vi "Tosca-Init Histogram.vi"(0 "Histogram":refnum<vi>, 7 "Results":T1[](array[typedef]), 11 "error in (no error)":errorcluster) -> (15 "error out":errorcluster)   [LabVIEW 2020]
uses:
  Classes/Parameters/Histogram Data.ctl
  <vilib>/Analysis/baseanly.llb/Mean (DBL).vi
  <vilib>/Analysis/NI_AALBase.lvlib
  Classes/Parameters/Parameters.lvclass
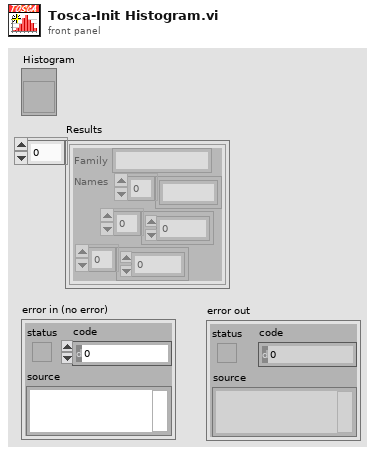
[diagram p1: front panel]
types:
  T1 = typedef "Parameters.lvclass/Histogram Data.ctl" = cluster{"Family":string, "Names":string[], "Colors":u32[], "N":i32[]}
  T2 = cluster{"Name":string, "Color":u32, "Style":u8, "Point Style":u8, "Name Visible":bool, "Allow Drag":bool, "Annotation Mode":u32, "Plot":i32, "Index":i32, "Position":cluster{"X":dbl, "Y":dbl}, "X Scale":u32, "Y Scale":u32, "Show Arrow":bool, "Lock Name":bool, "Plot Area":i32, "Label Offset":cluster{"X":dbl, "Y":dbl}}
  T3 = cluster{"Name":string, "Color":u32, "Style":u8, "Point Style":u8, "Name Visible":bool, "Allow Drag":bool, "Annotation Mode":u32, "Plot":i32, "Index":i32, "Position":cluster{"X":dbl, "Y":dbl}, "X Scale":u32, "Y Scale":u32, "Show Arrow":bool, "Lock Name":bool, "Plot Area":i32, "Label Offset":cluster{"X":dbl, "Y":dbl}}[]
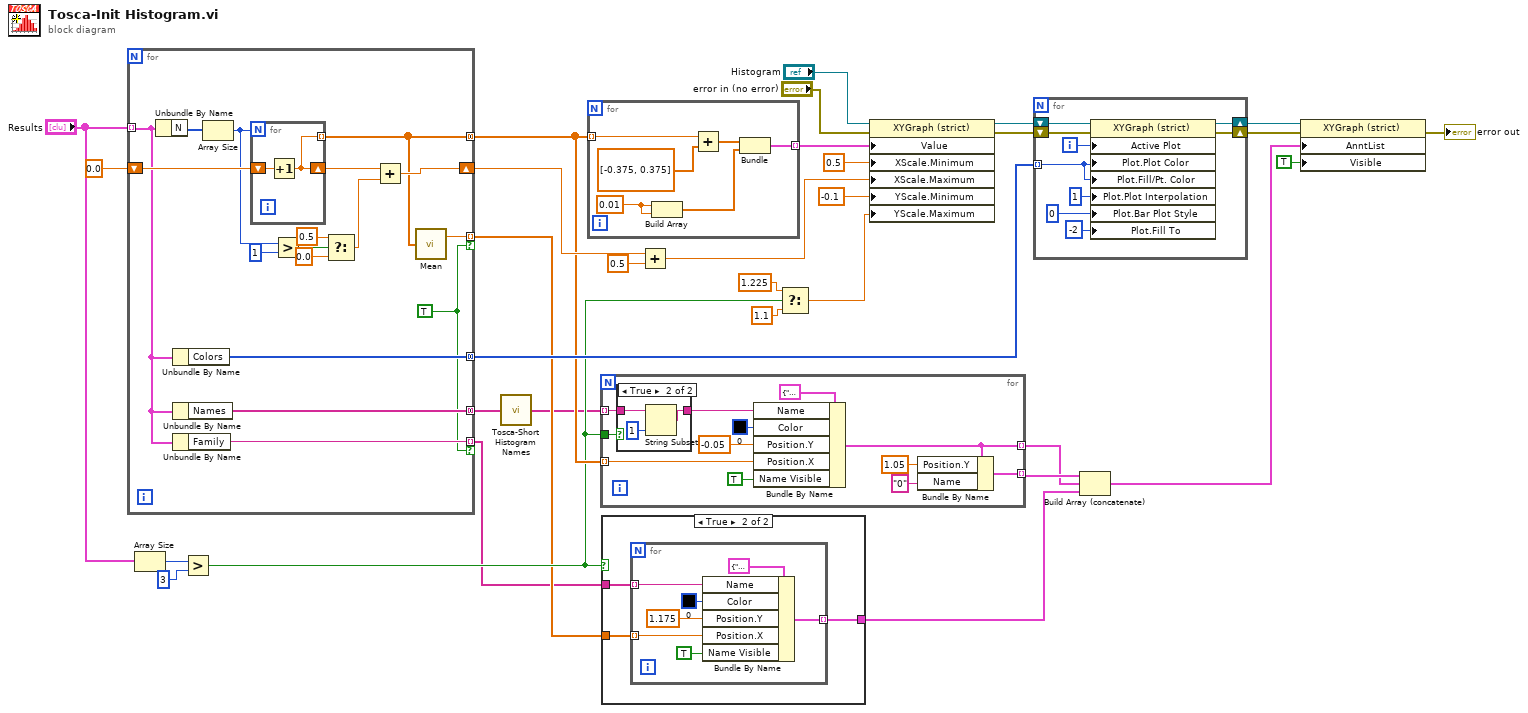
[diagram p0: block diagram]
diagram:
  n1 = for {
    tunnel: "Results" -> [w35] mode=indexing
    shift-right: [w47] -> w26
    shift-left: 0.0 -> [w49]
    tunnel: [w39] -> w15 mode=concatenating
    tunnel: [w36] -> w27 mode=concatenating
    tunnel: [w34] -> w2 mode=concatenating
    tunnel: [w37] -> w5 mode=indexing if=w33
    tunnel: [w38] -> w6 mode=indexing if=w33
    w33 = TRUE
    n2 = Unbundle By Name(w35) -> ("N"=w41:i32[])
    n3 = Unbundle By Name(w35) -> ("Colors"=w36:u32[])
    n4 = Unbundle By Name(w35) -> ("Names"=w34:string[])
    n5 = Unbundle By Name(w35) -> ("Family"=w37:string)
    n6 = Array Size(array=w41) -> (size(s)=w40:i32)
    n7 = for {
      N: w40 -> [_]
      tunnel: [w50] -> w39 mode=indexing
      shift-right: [w50] -> w48
      shift-left: w49 -> [w51]
      n8 = Increment(x=w51) -> (x+1=w50:dbl)
    }
    n9 = Greater?(x=w40, y=1) -> (0:w45:bool)
    n10 = Select(t=0.5, s=w45, f=0.0) -> (s? t:f=w43:dbl)
    n11 = Add(x=w48, y=w43) -> (x+y=w47:dbl)
    n12 = call-poly <vilib>:"Mean.vi"("X"=w39) -> ("mean"=w38:dbl)  [unwired: 1 out]
  }
  n13 = Array Size(array="Results") -> (size(s)=w21:i32)
  n14 = Greater?(x=w21, y=3) -> (0:w7:bool)
  n15 = call "Tosca-Short Histogram Names.vi"("Names"=w2) -> ("Short names"=w1:string[])  [unwired: 14 in]
  n16 = for {
    tunnel: w15 -> [w55] mode=indexing
    tunnel: [w57] -> w25 mode=indexing
    w53 = 0.01
    n17 = Build Array(w53, w53) -> (w56:dbl[])
    n18 = Add(x=w55, y=dbl[] [-0.375, 0.375]) -> (x+y=w54:dbl[])
    n19 = Bundle(w54, w56) -> (w57:cluster{dbl[], dbl[]})  [unwired: 1 in]
  }
  n20 = for {
    tunnel: w1 -> [w59] mode=indexing
    tunnel: [w66] -> w18 mode=indexing
    tunnel: [w65] -> w19 mode=indexing
    tunnel: w15 -> [w61] mode=indexing
    tunnel: w7 -> [w60]
    n21 = case shown="True" w60 {
      tunnel: w59 -> [w70 w73]
      tunnel: [w70 w71] -> w58
      frame False {
      }
      frame True {
        n22 = String Subset(string=w73, length (rest)=1 ("length (rest)")) -> (substring=w71:string)  [unwired: 1 in]
      }
    }
    n23 = Bundle By Name(cluster=T2 {"Name"="", "Color"=0, "Style"=0, "Point Style"=0, "Name Visible"=FALSE, "Allow Drag"=FALSE, "Annotation Mode"=0, "Plot"=0, "Index"=0, "Position"={"X"=0.0, "Y"=0.0}, "X Scale"=0, "Y Scale"=0, "Show Arrow"=FALSE, "Lock Name"=FALSE, "Plot Area"=0, "Label Offset"={"X"=0.0, "Y"=0.0}} ("element"), "Name"=w58, "Color"=u32 0, "Position.Y"=-0.05, "Position.X"=w61, "Name Visible"=TRUE) -> (w66:T2)
    n24 = Bundle By Name(cluster=w66, "Position.Y"=1.05, "Name"="0") -> (w65:T2)
  }
  n25 = case shown="True" w7 {
    tunnel: w6 -> [_ w75]
    tunnel: w5 -> [_ w76]
    tunnel: [_ w74] -> w4
    frame False {
    }
    frame True {
      n26 = for {
        tunnel: w76 -> [w79] mode=indexing
        tunnel: w75 -> [w78] mode=indexing
        tunnel: [w77] -> w74 mode=indexing
        n27 = Bundle By Name(cluster=T2 {"Name"="", "Color"=0, "Style"=0, "Point Style"=0, "Name Visible"=FALSE, "Allow Drag"=FALSE, "Annotation Mode"=0, "Plot"=0, "Index"=0, "Position"={"X"=0.0, "Y"=0.0}, "X Scale"=0, "Y Scale"=0, "Show Arrow"=FALSE, "Lock Name"=FALSE, "Plot Area"=0, "Label Offset"={"X"=0.0, "Y"=0.0}} ("element"), "Name"=w79, "Color"=u32 0, "Position.Y"=1.175, "Position.X"=w78, "Name Visible"=TRUE) -> (w77:T2)
      }
    }
  }
  n28 = Add(x=w26, y=0.5) -> (x+y=w24:dbl)
  n29 = Select(t=1.225 ("Y Scale.Range:Maximum"), s=w7, f=1.1 ("Y Scale.Range:Maximum")) -> (s? t:f=w12:dbl)
  n30 = property class="XYGraph (strict)"(reference="Histogram", error in="error in (no error)", "Value"=w25, "XScale.Minimum"=0.5 ("X Scale.Range:Minimum"), "XScale.Maximum"=w24, "YScale.Minimum"=-0.1 ("Y Scale.Range:Minimum"), "YScale.Maximum"=w12) -> (reference out=w29:refnum<vi>, error out=w10:errorcluster)
  n31 = for {
    tunnel: w27 -> [w87] mode=indexing
    shift-right: [w86] -> w17
    shift-left: w29 -> [w92]
    shift-right: [w84] -> w9
    shift-left: w10 -> [w85]
    i -> [w91]
    n32 = property class="XYGraph (strict)"(reference=w92, error in=w85, "Active Plot"=w91, "Plot.Plot Color"=w87, "Plot.Fill/Pt. Color"=w87, "Plot.Plot Interpolation"=u8 1, "Plot.Bar Plot Style"=u8 0, "Plot.Fill To"=i16 -2) -> (reference out=w86:refnum<vi>, error out=w84:errorcluster)
  }
  n33 = Build Array (concatenate)(w19, w18, w4) -> (w16:T3)
  n34 = property class="XYGraph (strict)"(reference=w17, error in=w9, "AnntList"=w16, "Visible"=TRUE) -> (error out=→"error out":errorcluster)  [unwired: 1 out]
